vi "Sample-Encoder conversion.vi"(6 "Encoder Position":i32, 7 "Step Window radius":i32, 10 "New Sample Number":i16, 11 "Encoder offset":i16) -> (1 "Encoder destination":i32, 2 "Within Range?":bool, 3 "Encoder distance to move":i32)   [LabVIEW 2015]
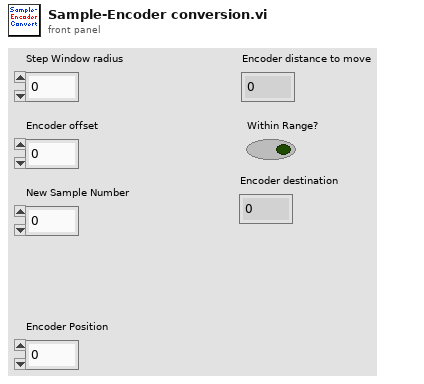
[diagram p1: front panel]
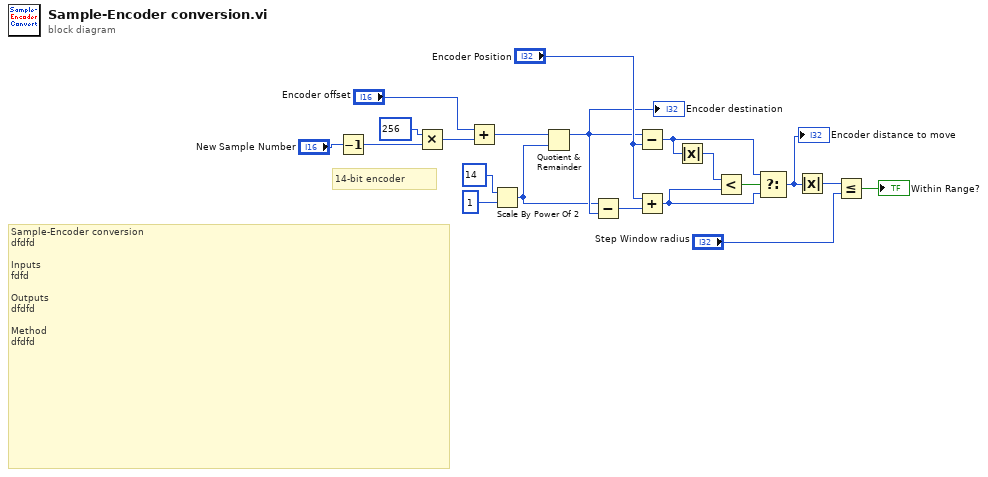
[diagram p0: block diagram]
diagram:
  # "Sample-Encoder conversion\ndfdfd\n\nInputs\nfdfd\n\nOutputs\ndfdfd\n\nMethod\ndfdfd"
  # "14-bit encoder"
  n1 = Decrement(x="New Sample Number") -> (x-1=w3:i16)
  n2 = Multiply(x=i16 256, y=w3) -> (x*y=w19:i16)
  n3 = Add(x="Encoder offset", y=w19) -> (x+y=w4:i16)
  n4 = Scale By Power Of 2(n=i16 14, x=i16 1) -> (x*2^n=w1:i16)
  n5 = Quotient & Remainder(x=w4, y=w1) -> (x-y*floor(x/y)=w2:i16)  [unwired: 1 out]
  "Encoder destination" <- w2
  n6 = Subtract(x=w1, y=w2) -> (x-y=w16:i16)
  n7 = Subtract(x=w2, y="Encoder Position") -> (x-y=w13:i32)
  n8 = Add(x="Encoder Position", y=w16) -> (x+y=w12:i32)
  n9 = Absolute Value(x=w13) -> (abs(x)=w15:i32)
  n10 = Less?(x=w15, y=w12) -> (x < y?=w14:bool)
  n11 = Select(t=w13, s=w14, f=w12) -> (s? t:f=w11:i32)
  "Encoder distance to move" <- w11
  n12 = Absolute Value(x=w11) -> (abs(x)=w10:i32)
  n13 = Less Or Equal?(x=w10, y="Step Window radius") -> (x <= y?=→"Within Range?":bool)
